vi "SwerveMath.vi"(0 "Inputs":dbl[](array[numeric]), 2 "Autonomous?":bool, 3 "Robot Centric?":bool=TRUE, 4 "Yaw":dbl) -> (20 "wheelSpeed1":dbl, 21 "wheelSpeed2":dbl, 22 "wheelSpeed3":dbl, 23 "wheelSpeed4":dbl, 24 "wheelAngle1":dbl, 25 "wheelAngle2":dbl, 26 "wheelAngle3":dbl, 27 "wheelAngle4":dbl)   [LabVIEW 2019]
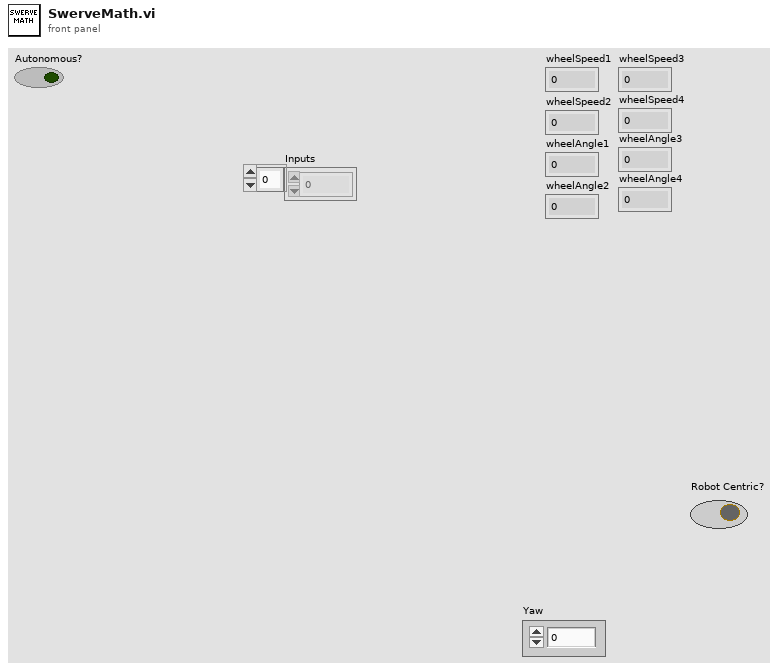
[diagram p1: front panel]
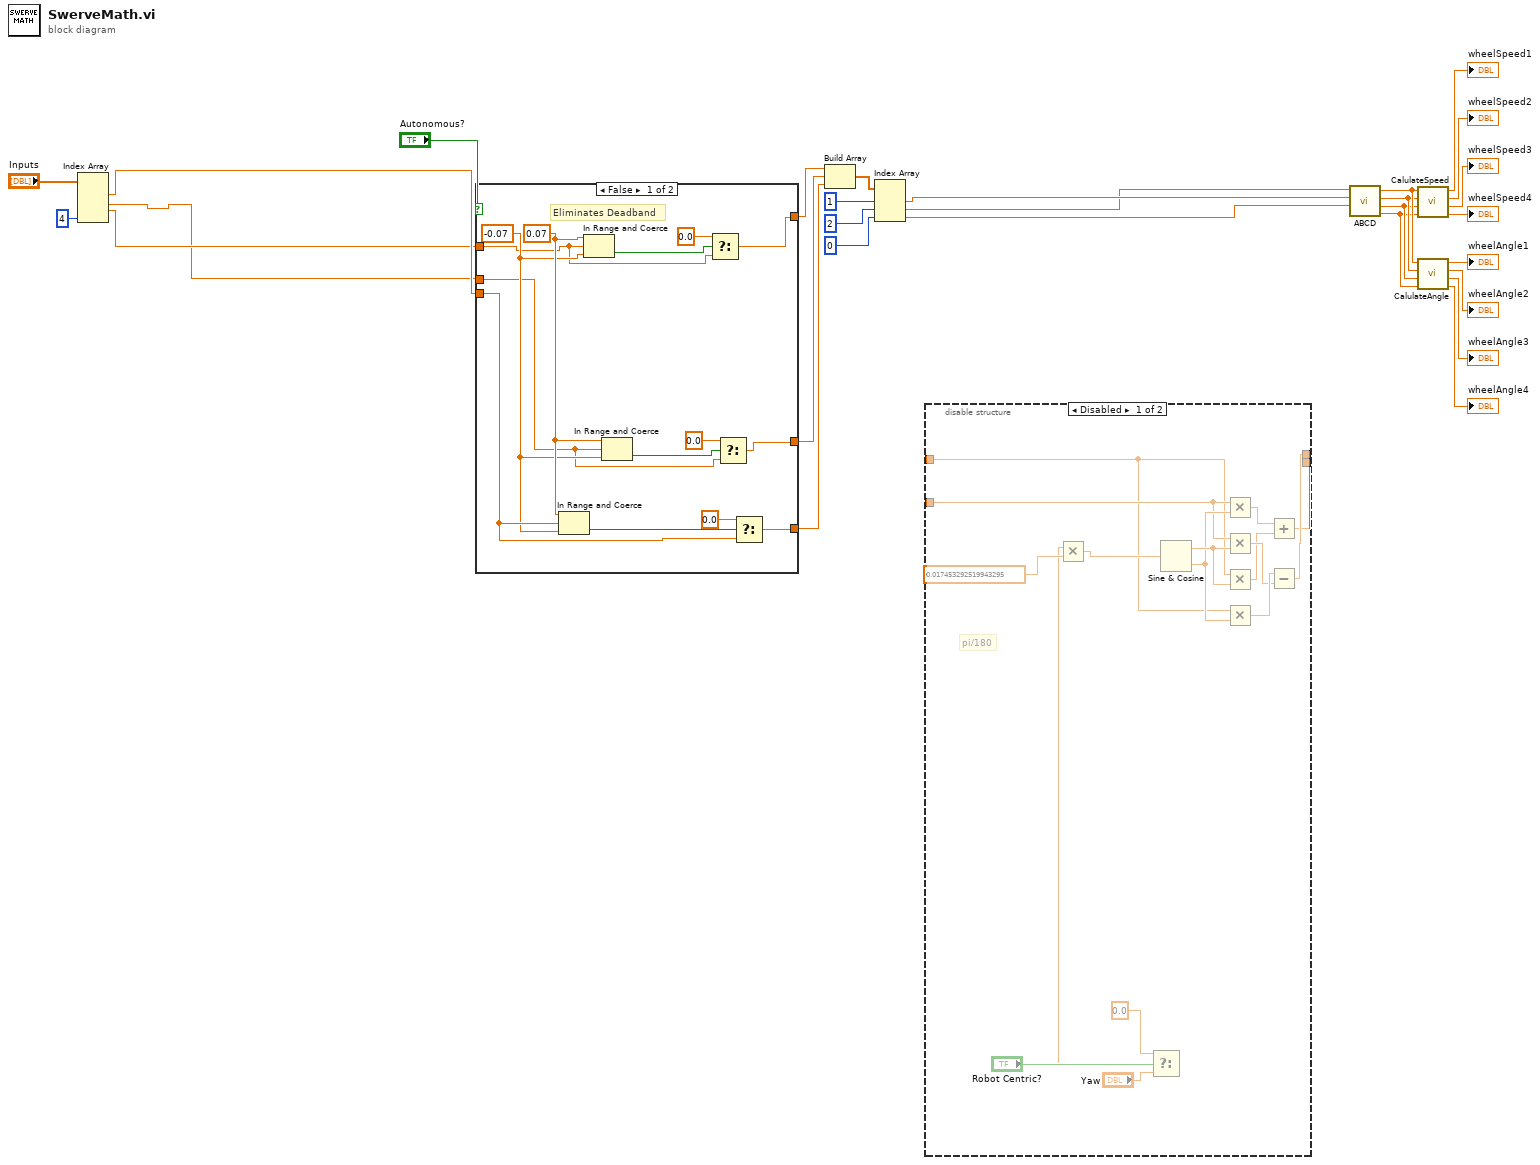
[diagram p0: block diagram]
diagram:
  n1 = Index Array(array="Inputs", index #4=4 ("index")) -> (element #1=w15:dbl, element #2=w1:dbl, element #3=w2:dbl)  [unwired: 3 in, 1 out]
  n2 = case shown="False" "Autonomous?" {
    tunnel: w1 -> [w31 w44]
    tunnel: w2 -> [w30 w45]
    tunnel: w15 -> [w41 w43]
    tunnel: [w36 w44] -> w8
    tunnel: [w29 w43] -> w7
    tunnel: [w37 w45] -> w6
    frame False {
      w32 = -0.07 ("lower limit")
      w33 = 0.07 ("upper limit")
      # "Eliminates Deadband"
      n3 = In Range and Coerce(upper limit=w33, x=w41, lower limit=w32) -> (In Range?=w42:bool)  [unwired: 1 out]
      n4 = In Range and Coerce(upper limit=w33, x=w30, lower limit=w32) -> (In Range?=w34:bool)  [unwired: 1 out]
      n5 = In Range and Coerce(upper limit=w33, x=w31, lower limit=w32) -> (In Range?=w35:bool)  [unwired: 1 out]
      n6 = Select(t=0.0, s=w34, f=w30) -> (s? t:f=w37:dbl)
      n7 = Select(t=0.0, s=w35, f=w31) -> (s? t:f=w36:dbl)
      n8 = Select(t=0.0, s=w42, f=w41) -> (s? t:f=w29:dbl)
    }
    frame True {
    }
  }
  n9 = Build Array(w6, w8, w7) -> (w9:dbl[])
  n10 = Index Array(array=w9, index #1=1 ("index"), index #2=2 ("index"), index #3=0 ("index")) -> (element #1=w5:dbl, element #2=w4:dbl, element #3=w10:dbl)
  n11 = disable-structure shown="Disabled" {
    disable-tunnel: _ -> [w49 _]
    disable-tunnel: _ -> [w48 _]
    disable-tunnel: [w47 _] -> _
    disable-tunnel: [w46 _] -> _
    frame Disabled {
      # "pi/180"
      n12 = Select(t=0.0, s="Robot Centric?", f="Yaw") -> (s? t:f=w51:dbl)
      n13 = Multiply(x=w51, y=0.017453292519943295) -> (x*y=w50:dbl)
      n14 = Sine & Cosine(0:w50) -> (1:w55:dbl, 2:w54:dbl)
      n15 = Multiply(x=w49, y=w54) -> (x*y=w53:dbl)
      n16 = Multiply(x=w49, y=w55) -> (x*y=w56:dbl)
      n17 = Multiply(x=w48, y=w55) -> (x*y=w52:dbl)
      n18 = Multiply(x=w48, y=w54) -> (x*y=w57:dbl)
      n19 = Add(x=w53, y=w52) -> (x+y=w46:dbl)
      n20 = Subtract(x=w57, y=w56) -> (x-y=w47:dbl)
    }
    frame Enabled {
    }
  }
  n21 = call "ABCD.vi"("z"=w10, "y"=w5, "x"=w4) -> ("D"=w24:dbl, "C"=w25:dbl, "B"=w26:dbl, "A"=w27:dbl)  [unwired: 5 in]
  n22 = call "CalulateSpeed.vi"("D"=w24, "C"=w25, "B"=w26, "A"=w27) -> ("wheelSpeed4"=→"wheelSpeed4":dbl, "wheelSpeed3"=→"wheelSpeed3":dbl, "wheelSpeed2"=→"wheelSpeed2":dbl, "wheelSpeed1"=→"wheelSpeed1":dbl)  [unwired: 4 in]
  n23 = call "CalulateAngle.vi"("D"=w24, "C"=w25, "B"=w26, "A"=w27) -> ("wheelAngle4"=→"wheelAngle4":dbl, "wheelAngle3"=→"wheelAngle3":dbl, "wheelAngle2"=→"wheelAngle2":dbl, "wheelAngle1"=→"wheelAngle1":dbl)  [unwired: 4 in]
